vi "HW3_圖片濾鏡.vi"() -> ()   [LabVIEW 2018]
uses:
  <vilib>/Utility/miscctls.llb/LVPoint32TypeDef.ctl
  <vilib>/Utility/miscctls.llb/LVBoundsTypeDef.ctl
panel:
  in  "Image Type":enum16{"JPG", "PNG", "BMP"}(ring)
  out "Coords":T1
  in  "img path":path
  out "B":u8
  out "G":u8
  out "R":u8
  in  "B":u8(slide) scale=0.0..255.0
  in  "G":u8(slide) scale=0.0..255.0
  in  "R":u8(slide) scale=0.0..255.0
  out "img out":picture
  out "org img":picture
  # "記得在這邊選擇圖片"
  # "調整RGB條後記得點擊一下圖片才會有濾鏡改變\n因為將圖片元件放在座標 (0, 0) 因此滑鼠點擊的座標會對應實際圖片座標"
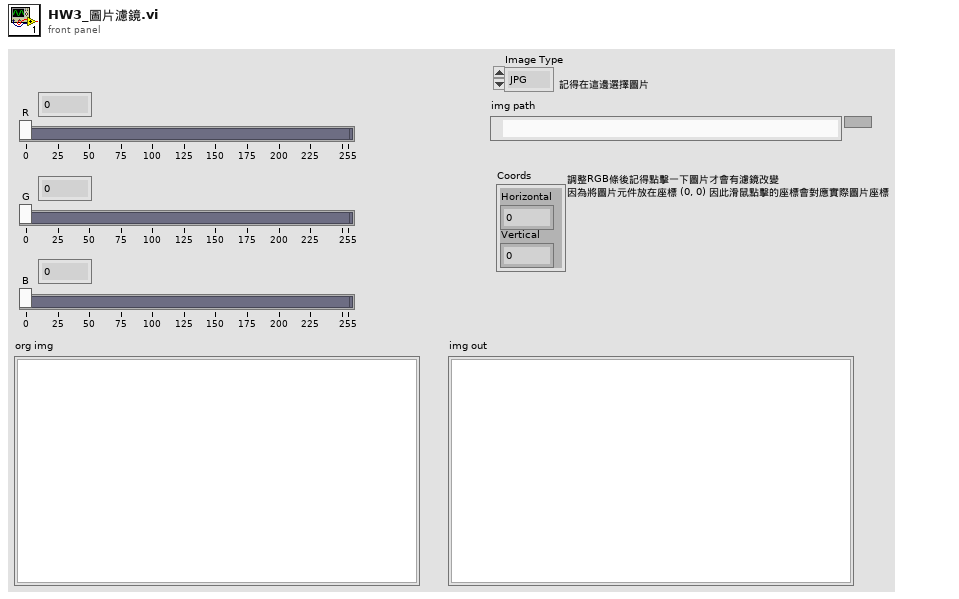
[diagram p1: front panel]
types:
  T1 = typedef "LVPoint32TypeDef.ctl" = cluster{"Horizontal":i32, "Vertical":i32}
  T2 = typedef "LVBoundsTypeDef.ctl" = cluster{"Width":u32, "Height":u32}
  T3 = typedef "imagedata.ctl" = cluster{"image type":i32, "image depth":i32, "image":u8[], "mask":u8[], "colors":u32[], "Rectangle":cluster{"left":i16, "top":i16, "right":i16, "bottom":i16}}
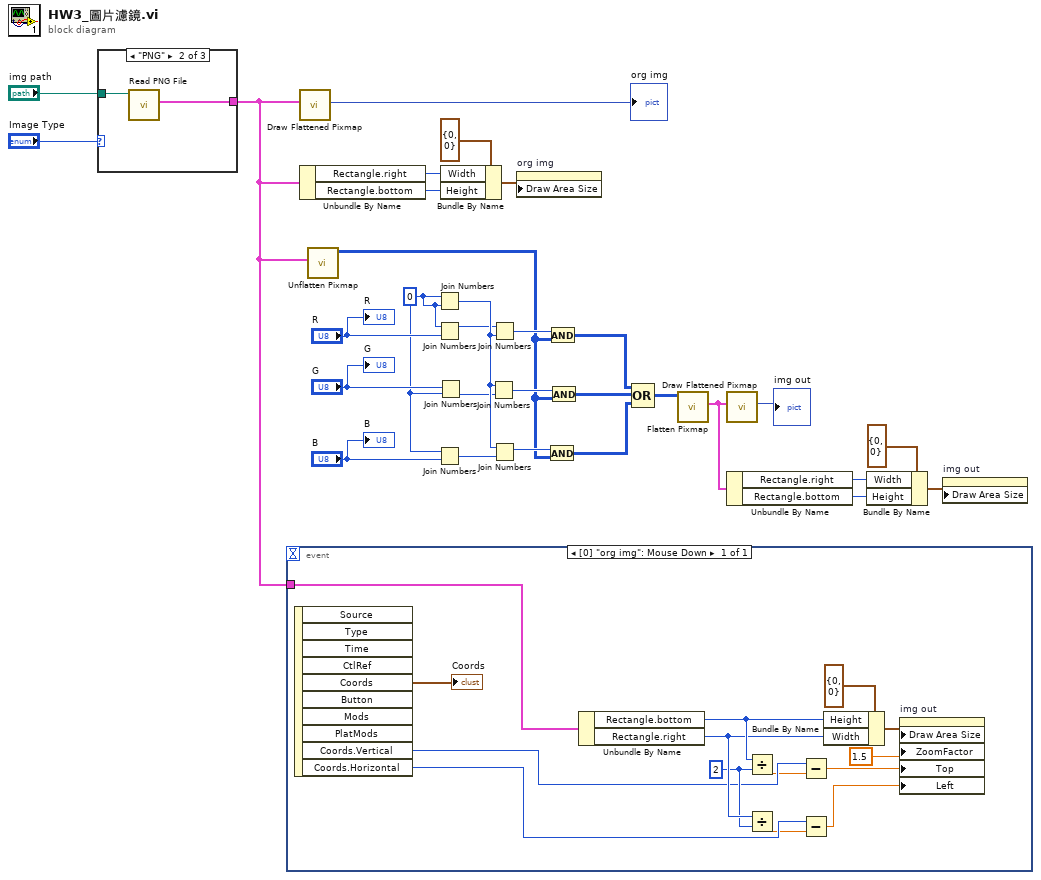
[diagram p0: block diagram]
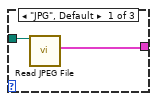
[diagram p2: hidden frame]
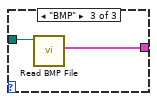
[diagram p3: hidden frame]
diagram:
  w6 = u8 0 ("hi")
  n1 = case shown="\"PNG\"" "Image Type" {
    tunnel: "img path" -> [w32 w34 w36]
    tunnel: [w31 w33 w35] -> w1
    frame "JPG", Default {
      n2 = call <vilib>:"Read JPEG File.vi"("path to JPEG file"=w32) -> ("image data"=w31:T3)  [unwired: 8 in, 2 out]
    }
    frame "PNG" {
      n3 = call <vilib>:"Read PNG File.vi"("path to PNG file"=w34) -> ("image data"=w33:T3)  [unwired: 8 in, 2 out]
    }
    frame "BMP" {
      n4 = call <vilib>:"Read BMP File.vi"("path to BMP file"=w36) -> ("image data"=w35:T3)  [unwired: 8 in, 2 out]
    }
  }
  n5 = event shown="[0] \"org img\": Mouse Down" {
    selector: _ -> [_]
    dyn-events: _ -> [_]
    timeout: _ -> [_]
    tunnel: w1 -> [w37]
    event "org img": Mouse Down {
      w44 = i16 2 ("y")
      n6 = event-data() -> ("Coords"=→"Coords":T1, "Coords.Vertical"=w40:i32, "Coords.Horizontal"=w41:i32)  [unwired: 1 in, 7 out]
      n7 = Unbundle By Name(w37) -> ("Rectangle.bottom"=w46:i16, "Rectangle.right"=w45:i16)
      n8 = Divide(x=w46, y=w44) -> (x/y=w39:dbl)
      n9 = Divide(x=w45, y=w44) -> (x/y=w38:dbl)
      n10 = Subtract(x=w40, y=w39) -> (x-y=w43:dbl)
      n11 = Subtract(x=w41, y=w38) -> (x-y=w42:dbl)
      n12 = Bundle By Name(cluster=T2 {"Width"=0, "Height"=0} ("Draw Area Size"), "Height"=w46, "Width"=w45) -> (w49:T2)
      n13 = property on="img out" class="Pict"("Draw Area Size"=w49, "ZoomFactor"=sgl 1.5 ("Zoom Factor"), "Top"=w43, "Left"=w42) -> ()  [unwired: 2 in, 2 out]
    }
  }
  n14 = call <vilib>:"Draw Flattened Pixmap.vi"("image data"=w1) -> ("new picture"=→"org img":picture)  [unwired: 8 in]
  n15 = Unbundle By Name(w1) -> ("Rectangle.right"=w27:i16, "Rectangle.bottom"=w26:i16)
  n16 = call <vilib>:"Unflatten Pixmap.vi"("image data"=w1) -> ("24-bit pixmap"=w10:u32[][])  [unwired: 4 in, 6 out]
  n17 = Join Numbers(hi=w6, lo=w6) -> ((hi.lo)=w17:u16)
  n18 = Join Numbers(hi=w6, lo="R") -> ((hi.lo)=w16:u16)
  n19 = Join Numbers(hi=w6, lo="B") -> ((hi.lo)=w13:u16)
  n20 = Join Numbers(hi="G", lo=w6) -> ((hi.lo)=w15:u16)
  n21 = Bundle By Name(cluster=T2 {"Width"=0, "Height"=0} ("Draw Area Size"), "Width"=w27, "Height"=w26) -> (w28:T2)
  n22 = Join Numbers(hi=w17, lo=w15) -> ((hi.lo)=w19:u32)
  n23 = Join Numbers(hi=w16, lo=w17) -> ((hi.lo)=w20:u32)
  n24 = Join Numbers(hi=w17, lo=w13) -> ((hi.lo)=w18:u32)
  n25 = property on="org img" class="Pict"("Draw Area Size"=w28) -> ()  [unwired: 2 in, 2 out]
  n26 = And(x=w18, y=w10) -> (x .and. y?=w23:u32[][])
  n27 = And(x=w20, y=w10) -> (x .and. y?=w11:u32[][])
  n28 = And(x=w19, y=w10) -> (x .and. y?=w24:u32[][])
  n29 = Compound Arithmetic op=OR(w11, w24, w23) -> (w22:u32[][])
  n30 = call <vilib>:"Flatten Pixmap.vi"("24-bit pixmap"=w22) -> ("image data"=w4:T3)  [unwired: 10 in]
  n31 = call <vilib>:"Draw Flattened Pixmap.vi"("image data"=w4) -> ("new picture"=→"img out":picture)  [unwired: 8 in]
  n32 = Unbundle By Name(w4) -> ("Rectangle.right"=w9:i16, "Rectangle.bottom"=w8:i16)
  n33 = Bundle By Name(cluster=T2 {"Width"=0, "Height"=0} ("Draw Area Size"), "Width"=w9, "Height"=w8) -> (w7:T2)
  n34 = property on="img out" class="Pict"("Draw Area Size"=w7) -> ()  [unwired: 2 in, 2 out]
  "R" <- "R"
  "G" <- "G"
  "B" <- "B"
